vi "ActionVIOnSave Check Errors.vi"(8 "error in (no error)":errorcluster, 11 "Device Item Ref in":T1 format="%.0x") -> (0 "error out":errorcluster, 3 "Device Item Ref out":T1 format="%.0x")   [LabVIEW 2019, in "Instrument Addon System Explorer.lvlib"]
uses:
  Instrument Addon System Explorer.lvlib
  <vilib>/NI VeriStand/Custom Device API/Custom Device Item Ref.ctl
  Addon Shared/Types/FG Control.ctl
  NationalInstruments.VeriStand.SystemStorage
  NationalInstruments.VeriStand
  Addon Shared/SubVIs/Constants.vi
  <vilib>/NI VeriStand/Custom Device Tools/Custom Device Utility Library/NI VeriStand - Search for All Items by GUID.vi
  <vilib>/NI VeriStand/Custom Device API/NI VeriStand - Get Item Property.vi
  <vilib>/NI VeriStand/Custom Device API/Get Item Property (U32).vi
  <vilib>/NI VeriStand/Custom Device API/Get Item Property (Double).vi
  <vilib>/NI VeriStand/Custom Device API/Get Item Property (Boolean).vi
  <vilib>/NI VeriStand/Custom Device API/Get Item Property (String).vi
  <vilib>/NI VeriStand/Custom Device API/NI VeriStand - Set Item Property.vi
  <vilib>/NI VeriStand/Custom Device API/Set Item Property (U32).vi
  <vilib>/NI VeriStand/Custom Device API/Set Item Property (Double).vi
  <vilib>/NI VeriStand/Custom Device API/Set Item Property (Boolean).vi
  <vilib>/NI VeriStand/Custom Device API/Set Item Property (String).vi
  <vilib>/NI VeriStand/Custom Device API/Get Item Property (String Array).vi
  <vilib>/NI VeriStand/Custom Device API/Set Item Property (String Array).vi
  <vilib>/NI VeriStand/Custom Device Tools/Custom Device Utility Library/Custom Device Utility Library.lvlib
  Addon Shared/Instrument Addon Shared.lvlib
  <vilib>/NI VeriStand/Custom Device API/Custom Device API.lvlib
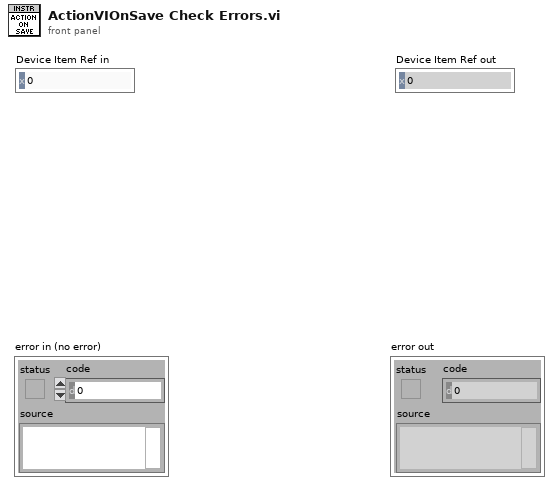
[diagram p1: front panel]
types:
  T1 = typedef "Custom Device API.lvlib/Custom Device Item Ref.ctl" = u64
  T2 = typedef "Instrument Addon Shared.lvlib/FG Control.ctl" = enum16{"Get", "Set"}
  T3 = typedef "Instrument Addon Shared.lvlib/Message Parameters.ctl" = cluster{"Generation Type":T4, "Period":dbl, "Include Protection":bool, "Type":string}
  T4 = typedef "Instrument Addon Shared.lvlib/Message Generation Type.ctl" = enum16{"Trigger Only", "Periodic & Trigger", "Value Change & Trigger"}
  T5 = typedef "Custom Device API.lvlib/Custom Device Pointer.ctl" = refnum<k24>
  T6 = typedef "Instrument Addon Shared.lvlib/Command Parameters.ctl" = cluster{"Command":string, "Linked Channels":T7[], "Pad":bool, "Length":u32, "Pad Value":u8}
  T7 = typedef "Instrument Addon Shared.lvlib/Linked Channel Cluster.ctl" = cluster{"Variable Name":string, "GUID":string}
  T8 = typedef "Instrument Addon Shared.lvlib/Response Parameters.ctl" = cluster{"Response":string, "Linked Channels":T7[], "Type Value":dbl, "Wait Type":T9, "Use Channel":bool, "Channel Path":string}
  T9 = typedef "Instrument Addon Shared.lvlib/Response Wait Type.ctl" = enum16{"Byte Count", "Wait sec"}
  T10 = typedef "Instrument Addon Shared.lvlib/Trigger Parameters.ctl" = cluster{"Use Channel":bool, "Channel Path":string}
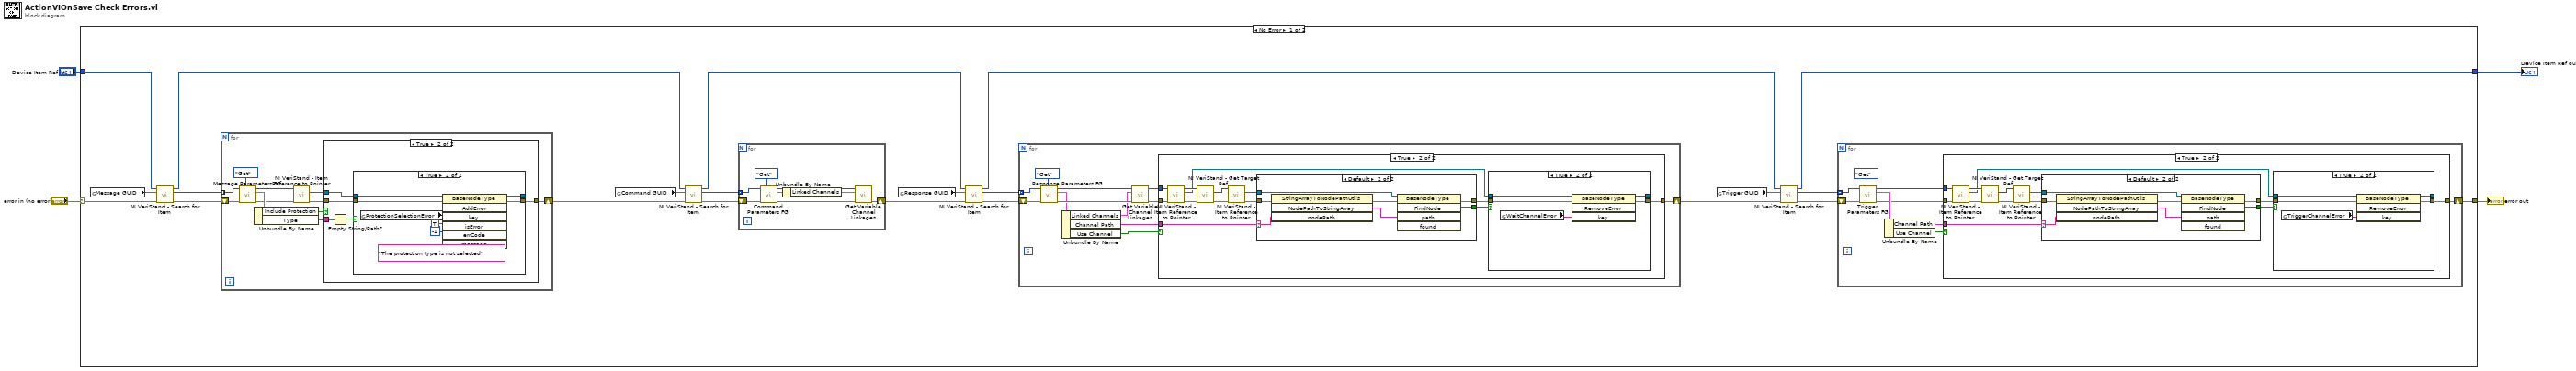
[diagram p0: block diagram]
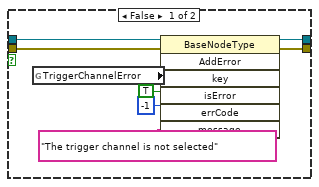
[diagram p3: hidden frame]
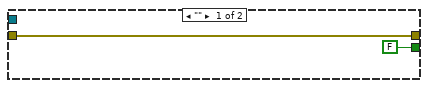
[diagram p4: hidden frame]
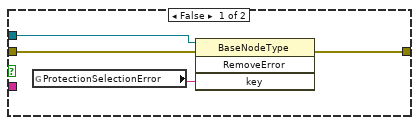
[diagram p5: hidden frame]
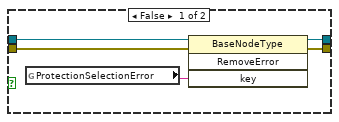
[diagram p6: hidden frame]
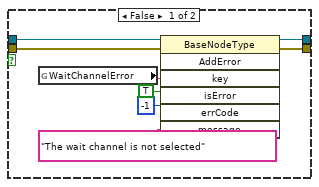
[diagram p8: hidden frame]
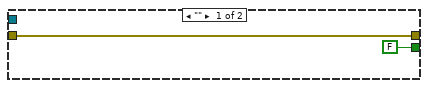
[diagram p9: hidden frame]
diagram:
  n1 = case shown="No Error" "error in (no error)" {
    selector: "error in (no error)" -> [w17 w162]
    tunnel: [w5 w162] -> w3
    tunnel: "Device Item Ref in" -> [w16 w161]
    tunnel: [w8 w161] -> w1
    frame No Error {
      n2 = global read "Constants.vi" "Message GUID"() -> (w18:string)
      n3 = call-poly <vilib>:"NI VeriStand - Search for Item.vi"("error in"=w17, "Item GUID"=w18, "Section Ref in"=w16) -> ("error out"=w13:errorcluster, "Item Refs"=w14:T1[], "Section Ref out"=w15:T1)  [unwired: 5 in, 1 out]
      n4 = for {
        tunnel: w14 -> [w82] mode=indexing
        shift-right: [w76] -> w12
        shift-left: w13 -> [w81]
        n5 = call "Message Parameters FG.vi"("Action"=FG_Control."Get", "error in (no error)"=w81, "Item Ref in"=w82) -> ("error out"=w75:errorcluster, "Message Settings out"=w79:T3, "Item Ref out"=w73:T1)  [unwired: 6 in]
        n6 = Unbundle By Name(w79) -> ("Include Protection"=w78:bool, "Type"=w77:string)
        n7 = call <vilib>:"NI VeriStand - Item Reference to Pointer.vi"("error in (no error)"=w75, "Item Ref in"=w73) -> ("error out"=w74:errorcluster, "Node Pointer"=w72:T5)  [unwired: 6 in, 2 out]
        n8 = case shown="True" w78 {
          tunnel: w77 -> [_ w91]
          tunnel: w74 -> [w84 w87]
          tunnel: w72 -> [w85 w88]
          tunnel: [w83 w89] -> w76
          frame False {
            n9 = global read "Constants.vi" "ProtectionSelectionError"() -> (w86:string)
            n10 = invoke class="BaseNodeType" method="RemoveError"(reference=w85, error in=w84, "key"=w86) -> (error out=w83:errorcluster)  [unwired: 1 in, 3 out]
          }
          frame True {
            n11 = Empty String/Path?(string/path=w91) -> (empty?=w90:bool)
            n12 = case shown="True" w90 {
              tunnel: w87 -> [w94 w100]
              tunnel: [w93 w104] -> w89
              tunnel: w88 -> [w96 w101]
              tunnel: [w95 w98] -> _
              frame False {
                n13 = global read "Constants.vi" "ProtectionSelectionError"() -> (w92:string)
                n14 = invoke class="BaseNodeType" method="RemoveError"(reference=w96, error in=w94, "key"=w92) -> (reference out=w95:T5, error out=w93:errorcluster)  [unwired: 1 in, 2 out]
              }
              frame True {
                n15 = global read "Constants.vi" "ProtectionSelectionError"() -> (w97:string)
                n16 = invoke class="BaseNodeType" method="AddError"(reference=w101, error in=w100, "key"=w97, "isError"=TRUE, "errCode"=-1, "message"="The protection type is not selected") -> (reference out=w98:T5, error out=w104:errorcluster)  [unwired: 1 in, 5 out]
              }
            }
          }
        }
      }
      n17 = global read "Constants.vi" "Command GUID"() -> (w26:string)
      n18 = call-poly <vilib>:"NI VeriStand - Search for Item.vi"("error in"=w12, "Item GUID"=w26, "Section Ref in"=w15) -> ("error out"=w25:errorcluster, "Item Refs"=w24:T1[], "Section Ref out"=w19:T1)  [unwired: 5 in, 1 out]
      n19 = for {
        tunnel: w24 -> [w156] mode=indexing
        shift-right: [w153] -> w20
        shift-left: w25 -> [w157]
        n20 = call "Command Parameters FG.vi"("Action"=FG_Control."Get", "error in (no error)"=w157, "Item Ref in"=w156) -> ("error out"=w159:errorcluster, "Command Parameters"=w155:T6, "Item Ref out"=w160:T1)  [unwired: 6 in]
        n21 = Unbundle By Name(w155) -> ("Linked Channels"=w154:T7[])
        n22 = call "Get Variable Channel Linkages.vi"("error in (no error)"=w159, "Linked Channels"=w154, "Item Ref in"=w160) -> ("error out"=w153:errorcluster)  [unwired: 6 in, 2 out]
      }
      n23 = global read "Constants.vi" "Response GUID"() -> (w21:string)
      n24 = call-poly <vilib>:"NI VeriStand - Search for Item.vi"("error in"=w20, "Item GUID"=w21, "Section Ref in"=w19) -> ("error out"=w22:errorcluster, "Item Refs"=w23:T1[], "Section Ref out"=w9:T1)  [unwired: 5 in, 1 out]
      n25 = for {
        tunnel: w23 -> [w112] mode=indexing
        shift-right: [w105] -> w10
        shift-left: w22 -> [w113]
        n26 = call "Response Parameters FG.vi"("Action"=FG_Control."Get", "error in (no error)"=w113, "Item Ref in"=w112) -> ("error out"=w115:errorcluster, "Response Parameters"=w111:T8, "Item Ref out"=w116:T1)  [unwired: 6 in]
        n27 = Unbundle By Name(w111) -> ("Linked Channels"=w110:T7[], "Channel Path"=w107:string, "Use Channel"=w109:bool)
        n28 = call "Get Variable Channel Linkages.vi"("error in (no error)"=w115, "Linked Channels"=w110, "Item Ref in"=w116) -> ("error out"=w108:errorcluster, "Item Ref out"=w106:T1)  [unwired: 6 in, 1 out]
        n29 = case shown="True" w109 {
          tunnel: w108 -> [w117 w124]
          tunnel: w107 -> [_ w118]
          tunnel: w106 -> [_ w122]
          tunnel: [w117 w119] -> w105
          frame False {
          }
          frame True {
            n30 = call <vilib>:"NI VeriStand - Item Reference to Pointer.vi"("error in (no error)"=w124, "Item Ref in"=w122) -> ("error out"=w123:errorcluster, "Node Pointer"=w120:T5, "Item Ref out"=w121:T1)  [unwired: 6 in, 1 out]
            n31 = call <vilib>:"NI VeriStand - Get Target Ref.vi"("error in"=w123, "Item Ref in"=w121) -> ("error out"=w130:errorcluster, "Target Ref"=w129:T1)  [unwired: 6 in, 2 out]
            n32 = call <vilib>:"NI VeriStand - Item Reference to Pointer.vi"("error in (no error)"=w130, "Item Ref in"=w129) -> ("error out"=w128:errorcluster, "Node Pointer"=w127:T5)  [unwired: 6 in, 2 out]
            n33 = case shown="Default" w118 {
              selector: w118 -> [_ w147]
              tunnel: [w145 w152] -> w126
              tunnel: w128 -> [w145 w150]
              tunnel: w127 -> [_ w149]
              tunnel: [FALSE ("FindNode") w148] -> w125
              frame "" {
              }
              frame Default {
                n34 = invoke class="StringArrayToNodePathUtils" method="NodePathToStringArray"(error in=w150, "nodePath"=w147) -> (error out=w151:errorcluster, "NodePathToStringArray"=w146:string[])  [unwired: 2 in, 2 out]
                n35 = invoke class="BaseNodeType" method="FindNode"(reference=w149, error in=w151, "path"=w146) -> (error out=w152:errorcluster, "FindNode"=w148:bool)  [unwired: 2 in, 3 out]
              }
            }
            n36 = case shown="True" w125 {
              tunnel: w126 -> [w134 w141]
              tunnel: [w138 w140] -> w119
              tunnel: w120 -> [w135 w143]
              tunnel: [w132 w142] -> _
              frame False {
                n37 = global read "Constants.vi" "WaitChannelError"() -> (w131:string)
                n38 = invoke class="BaseNodeType" method="AddError"(reference=w135, error in=w134, "key"=w131, "isError"=TRUE, "errCode"=-1, "message"="The wait channel is not selected") -> (reference out=w132:T5, error out=w138:errorcluster)  [unwired: 1 in, 5 out]
              }
              frame True {
                n39 = global read "Constants.vi" "WaitChannelError"() -> (w139:string)
                n40 = invoke class="BaseNodeType" method="RemoveError"(reference=w143, error in=w141, "key"=w139) -> (reference out=w142:T5, error out=w140:errorcluster)  [unwired: 1 in, 2 out]
              }
            }
          }
        }
      }
      n41 = global read "Constants.vi" "Trigger GUID"() -> (w11:string)
      n42 = call-poly <vilib>:"NI VeriStand - Search for Item.vi"("error in"=w10, "Item GUID"=w11, "Section Ref in"=w9) -> ("error out"=w6:errorcluster, "Item Refs"=w7:T1[], "Section Ref out"=w8:T1)  [unwired: 5 in, 1 out]
      n43 = for {
        tunnel: w7 -> [w33] mode=indexing
        shift-right: [w27] -> w5
        shift-left: w6 -> [w34]
        n44 = call "Trigger Parameters FG.vi"("Action"=FG_Control."Get", "error in (no error)"=w34, "Item Ref in"=w33) -> ("error out"=w29:errorcluster, "Trigger Parameters"=w32:T10, "Item Ref out"=w28:T1)  [unwired: 6 in]
        n45 = Unbundle By Name(w32) -> ("Channel Path"=w30:string, "Use Channel"=w31:bool)
        n46 = case shown="True" w31 {
          tunnel: w29 -> [w36 w43]
          tunnel: w30 -> [_ w37]
          tunnel: w28 -> [_ w41]
          tunnel: [w36 w38] -> w27
          frame False {
          }
          frame True {
            n47 = call <vilib>:"NI VeriStand - Item Reference to Pointer.vi"("error in (no error)"=w43, "Item Ref in"=w41) -> ("error out"=w42:errorcluster, "Node Pointer"=w39:T5, "Item Ref out"=w40:T1)  [unwired: 6 in, 1 out]
            n48 = call <vilib>:"NI VeriStand - Get Target Ref.vi"("error in"=w42, "Item Ref in"=w40) -> ("error out"=w49:errorcluster, "Target Ref"=w48:T1)  [unwired: 6 in, 2 out]
            n49 = call <vilib>:"NI VeriStand - Item Reference to Pointer.vi"("error in (no error)"=w49, "Item Ref in"=w48) -> ("error out"=w47:errorcluster, "Node Pointer"=w46:T5)  [unwired: 6 in, 2 out]
            n50 = case shown="Default" w37 {
              selector: w37 -> [_ w66]
              tunnel: [w64 w71] -> w45
              tunnel: w47 -> [w64 w69]
              tunnel: w46 -> [_ w68]
              tunnel: [FALSE ("FindNode") w67] -> w44
              frame "" {
              }
              frame Default {
                n51 = invoke class="StringArrayToNodePathUtils" method="NodePathToStringArray"(error in=w69, "nodePath"=w66) -> (error out=w70:errorcluster, "NodePathToStringArray"=w65:string[])  [unwired: 2 in, 2 out]
                n52 = invoke class="BaseNodeType" method="FindNode"(reference=w68, error in=w70, "path"=w65) -> (error out=w71:errorcluster, "FindNode"=w67:bool)  [unwired: 2 in, 3 out]
              }
            }
            n53 = case shown="True" w44 {
              tunnel: w45 -> [w53 w60]
              tunnel: [w57 w59] -> w38
              tunnel: w39 -> [w54 w62]
              tunnel: [w51 w61] -> _
              frame False {
                n54 = global read "Constants.vi" "TriggerChannelError"() -> (w50:string)
                n55 = invoke class="BaseNodeType" method="AddError"(reference=w54, error in=w53, "key"=w50, "isError"=TRUE, "errCode"=-1, "message"="The trigger channel is not selected") -> (reference out=w51:T5, error out=w57:errorcluster)  [unwired: 1 in, 5 out]
              }
              frame True {
                n56 = global read "Constants.vi" "TriggerChannelError"() -> (w58:string)
                n57 = invoke class="BaseNodeType" method="RemoveError"(reference=w62, error in=w60, "key"=w58) -> (reference out=w61:T5, error out=w59:errorcluster)  [unwired: 1 in, 2 out]
              }
            }
          }
        }
      }
    }
    frame Error {
    }
  }
  "error out" <- w3
  "Device Item Ref out" <- w1
